vi "Accelerator Pedal Simulation.vi"(9 "stop":bool, 10 "Accelerate":bool) -> (3 "Meter":i32(knob) scale=0.0..100.0)   [LabVIEW 2020]
doc: "This Simple VI will be a kind of demonstration of Accelerator Pedal of Automobile.\n\nGuide for this VI:\n\n1) Run the VI.\n2) Press and Hold the Pedal (PUSH) by right clicking your mouse button and Hold it like you hold the Accelerator in real world.\n3) Release the PUSH button and you will see Speed Gradually decreasing.\n4) Press and Hold PUSH button again to increase the Speed.\n5) Press STOP button to end the Simulation."
panel:
  out "Car ON?":bool
  # "Speed in Km/hr"
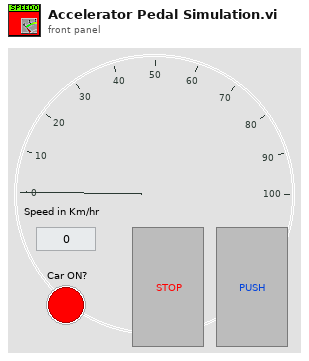
[diagram p1: front panel]
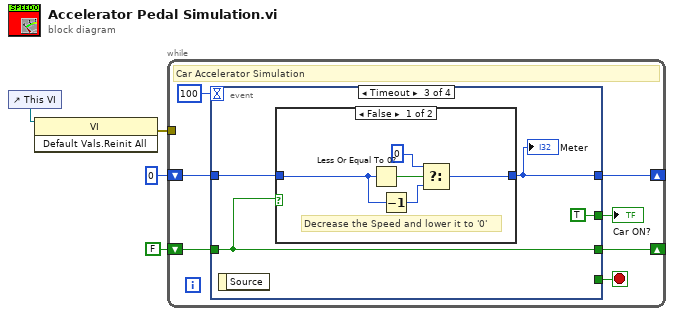
[diagram p0: block diagram]
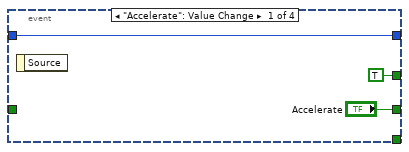
[diagram p2: hidden frame]
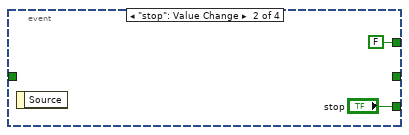
[diagram p3: hidden frame]
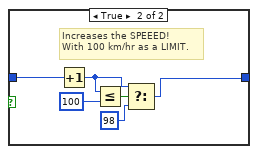
[diagram p4: hidden frame]
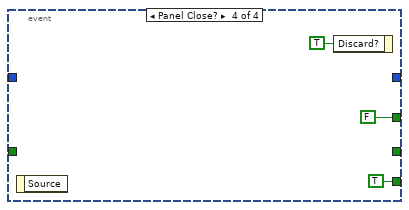
[diagram p5: hidden frame]
diagram:
  n1 = control-ref of="This VI"() -> (w1:refnum<vi>)
  n2 = invoke class="VI" method="Default Vals.Reinit All"(reference=w1) -> (error out=w2:errorcluster)  [unwired: 2 in, 2 out]
  n3 = while {
    shift-right: [w10] -> _
    shift-left: 0 -> [w11]
    shift-right: [w6] -> _
    shift-left: FALSE -> [w7]
    tunnel: w2 -> [_]
    stop <- w9 stop-if-true
    # "Car Accelerator Simulation"
    n4 = event shown="[2] Timeout" {
      selector: _ -> [_ _ _ _]
      dyn-events: _ -> [_ _ _ _]
      timeout: 100 -> [_ _ _ _]
      tunnel: w11 -> [w14 _ w20 _]
      tunnel: [w14 _ w19 _] -> w10
      tunnel: [_ "stop" _ TRUE ("stop")] -> w9
      tunnel: w7 -> [_ _ w18 _]
      tunnel: ["Accelerate" _ w18 _] -> w6
      tunnel: [TRUE ("stop") FALSE ("stop") TRUE ("stop") FALSE ("stop")] -> w5
      event "Accelerate": Value Change {
        n5 = event-data() -> ()  [unwired: 1 in, 1 out]
      }
      event "stop": Value Change {
        n6 = event-data() -> ()  [unwired: 1 in, 1 out]
      }
      event Timeout {
        n7 = event-data() -> ()  [unwired: 1 in, 1 out]
        n8 = case shown="False" w18 {
          tunnel: w20 -> [w25 w31]
          tunnel: [w24 w28] -> w19
          frame False {
            # "Decrease the Speed and lower it to '0'"
            n9 = Less Or Equal To 0?(x=w25) -> (x <= 0?=w23:bool)
            n10 = Decrement(x=w25) -> (x-1=w21:i32)
            n11 = Select(t=0, s=w23, f=w21) -> (s? t:f=w24:i32)
          }
          frame True {
            # "Increases the SPEEED! \nWith 100 km/hr as a LIMIT."
            n12 = Increment(x=w31) -> (x+1=w29:i32)
            n13 = Less Or Equal?(x=w29, y=100) -> (x <= y?=w30:bool)
            n14 = Select(t=w29, s=w30, f=98) -> (s? t:f=w28:i32)
          }
        }
        "Meter" <- w19
      }
      event Panel Close? {
        n15 = event-data() -> ()  [unwired: 1 in, 1 out]
        n16 = event-data("Discard?"=TRUE) -> ()  [unwired: 1 in, 1 out]
      }
    }
    "Car ON?" <- w5
  }
